vi "Get Control Value and DefValue.vi"(8 "错误输入（无错误）":errorcluster, 9 "Mode":enum16{"Get Value", "Get DefValue"}(ring), 11 "Ctl Ref In":refnum<vi>) -> (0 "错误输出":errorcluster, 1 "Value":variant, 2 "Type Enum":T1, 3 "Ctl Ref Out":refnum<vi>, 5 "Name":string)   [LabVIEW 2012, in "CtrlRef.lvlib"]
uses:
  CtrlRef.lvlib
  <vilib>/Utility/VariantDataType/Type.ctl
  <vilib>/Utility/VariantDataType/VariantType.lvlib
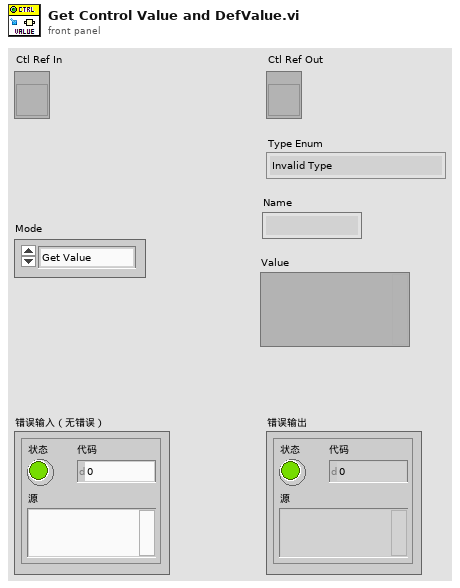
[diagram p1: front panel]
types:
  T1 = typedef "VariantType.lvlib/Type.ctl" = enum8{"Invalid Type", "Void", "I8", "I16", "I32", "I64", "U8", "U16", "U32", "U64", "Single Float", "Double Float", "Extended Float", "Single Complex", "Double Complex", "Extended Complex", "Enum U8", "Enum U16", "Enum U32", "Enum U64", "Single Float With Unit", "Double Float With Unit", "Extended Float With Unit", "Single Complex with Unit", "Double Complex with Unit", "Extended Complex with Unit", "Boolean", "String", "Path", "Picture", "Tag", "Array", "Cluster", "Variant", "LV Variant", "Waveform", "Timestamp", "Digital Waveform", "Digital Data", "ExpressData", "Refnum", "External Data", "VI", "Poly VI", "LabVIEW Class Instance", "Fixed Point"}
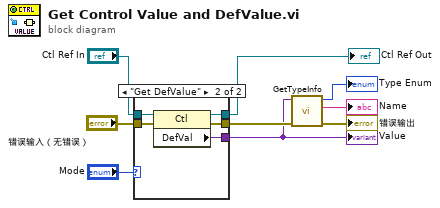
[diagram p0: block diagram]
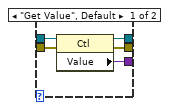
[diagram p2: hidden frame]
diagram:
  n1 = case shown="\"Get DefValue\"" "Mode" {
    tunnel: "错误输入（无错误）" -> [w14 w19]
    tunnel: "Ctl Ref In" -> [w13 w18]
    tunnel: [w12 w17] -> w6
    tunnel: [w11 w16] -> w4
    tunnel: [w10 w15] -> w3
    frame "Get Value", Default {
      n2 = property class="Ctl"(reference=w13, error in=w14) -> (reference out=w12:refnum<vi>, error out=w11:errorcluster, "Value"=w10:variant)
    }
    frame "Get DefValue" {
      n3 = property class="Ctl"(reference=w18, error in=w19) -> (reference out=w17:refnum<vi>, error out=w16:errorcluster, "DefVal"=w15:variant)
    }
  }
  "Ctl Ref Out" <- w6
  "Value" <- w3
  n4 = call <vilib>:"GetTypeInfo.vi"("error in (no error)"=w4, "Variant"=w3) -> ("error out"=→"错误输出":errorcluster, "Name"=→"Name":string, "Type Enum"=→"Type Enum":T1)  [unwired: 5 in, 2 out]
